vi "TestPlotBoat.vi"() -> ()   [LabVIEW 2013]
uses:
  cRIO_Code/Data/TypeDefs/UTM Location.ctl
panel:
  in  "Map":enum16{"Grid"}(ring)
  in  "Trace Path":bool=TRUE
  out "Boat Outside Img":bool
  in  "Heading":dbl
  in  "stop":bool
  in  "UTM boat location":T1={"UTM Zone"=0.0, "Hemisphere"=enum."North", "East"=1.0, "North"=1.0} {"North" format="%#_10f"; "East" format="%#_8f"}
  out "Mission Map":T2(plugin-control)
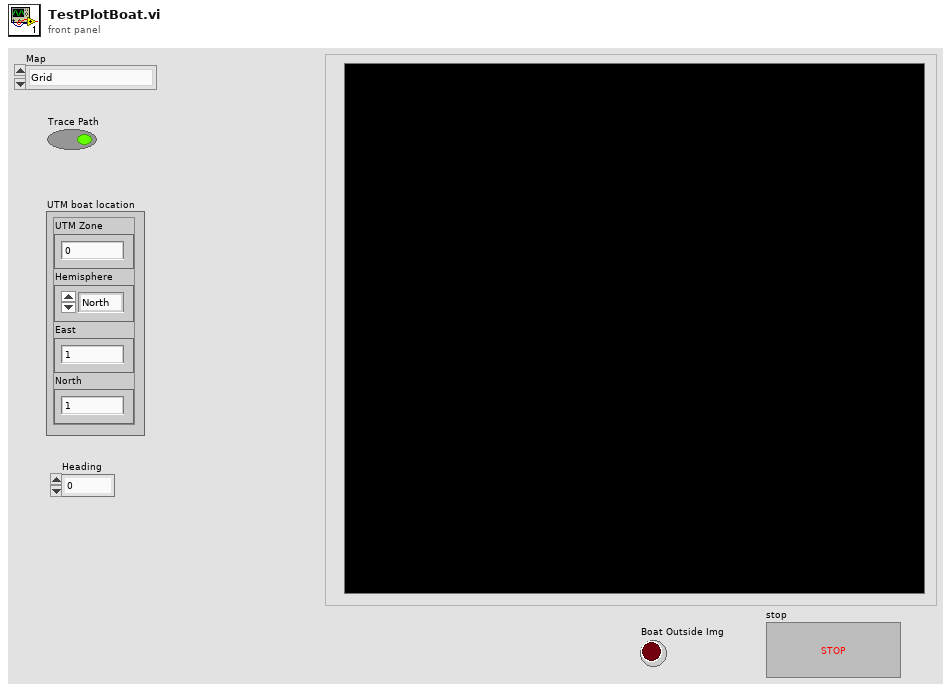
[diagram p1: front panel]
types:
  T1 = typedef "UTM Location.ctl" = cluster{"UTM Zone":dbl, "Hemisphere":enum16{"North", "South"}, "East":dbl, "North":dbl}
  T2 = typedef "IMAQ Image.ctl" = refnum<image>
  T3 = typedef "MapDistanceInfo.ctl" = cluster{"Meters/pixel":dbl, "Top Left Pixel UTM":T1, "Bottom Right Pixel UTM":T1}
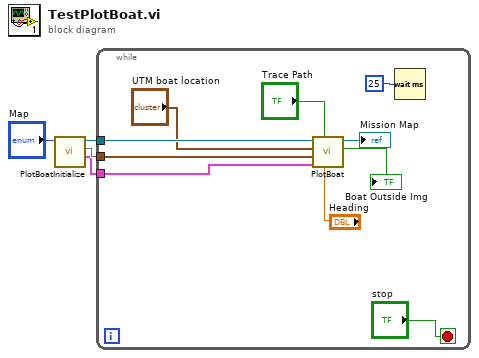
[diagram p0: block diagram]
diagram:
  n1 = call "PlotBoatInitialize.vi"("Map"="Map") -> ("MapDistanceInfo"=w2:T3, 2:w3, "Map Image Out"=w4:T2)  [unwired: 8 in]
  n2 = while {
    tunnel: w4 -> [w14]
    tunnel: w3 -> [w7]
    tunnel: w2 -> [w6]
    stop <- "stop" stop-if-true
    n3 = call "PlotBoat.vi"("Sail Setpoints"="Heading", "Trace Path"="Trace Path", "Heading"=w6, "MapDistanceInfo"=w7, "UTM Location"="UTM boat location", "Map in"=w14) -> ("Boat Outside Img"=→"Boat Outside Img":bool, "Map Out"=→"Mission Map":T2)  [unwired: 4 in]
    n4 = Wait (ms)(milliseconds to wait=u32 25) -> ()  [unwired: 1 out]
  }
